vi "File.Make Name Safe for Folder or File.vi"(3 "File Name":string) -> (1 "Fixed Name":string)   [LabVIEW 2024, in "EQMF.lvlib" / "File Utils.lvlib"]
doc: "This VI removes the extension from a file name.\n\nEXAMPLE:\n Input file name \"ABCD.txt\" will output \"ABCD\""
uses:
  File Utils.lvlib
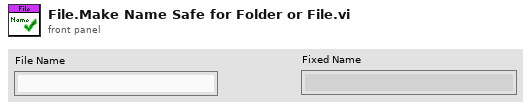
[diagram p1: front panel]
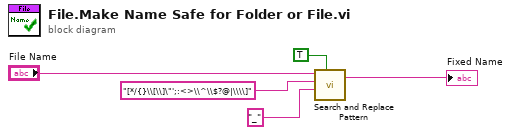
[diagram p0: block diagram]
diagram:
  n1 = call <vilib>:"Search and Replace Pattern.vi"("string"="File Name", "regular expression (\"\")"="[*/{}\\[\\]\"';:<>\\^\\$?@|\\\\]" ("regular expression (\"\")"), "replace string (\"\")"="_" ("regular expression (\"\")"), "replace all? (F)"=TRUE) -> ("result string"=→"Fixed Name":string)  [unwired: 1 in, 1 out]
